vi "周围雷数.vi"(9 "列":dbl, 10 "行":dbl, 11 "雷区":dbl[][](array[numeric])) -> (3 "雷数":dbl)   [LabVIEW 2012]
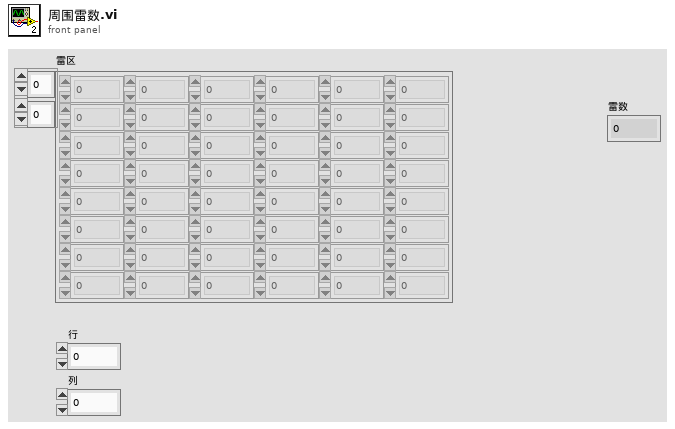
[diagram p1: front panel]
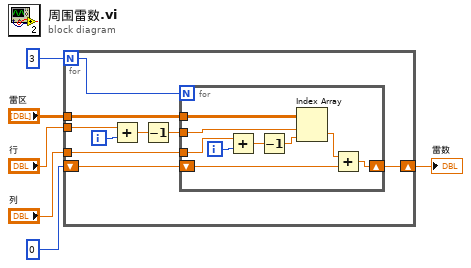
[diagram p0: block diagram]
diagram:
  n1 = for {
    N: 3 -> [w15]
    tunnel: "雷区" -> [w14]
    shift-right: [w7] -> w3
    shift-left: 0 -> [w13]
    tunnel: "行" -> [w10]
    tunnel: "列" -> [w12]
    i -> [w11]
    n2 = Add(x=w10, y=w11) -> (x+y=w9:dbl)
    n3 = Decrement(x=w9) -> (x-1=w8:dbl)
    n4 = for {
      N: w15 -> [_]
      tunnel: w14 -> [w21]
      shift-right: [w16] -> w7
      shift-left: w13 -> [w17]
      tunnel: w12 -> [w24]
      tunnel: w8 -> [w20]
      i -> [w23]
      n5 = Add(x=w24, y=w23) -> (x+y=w22:dbl)
      n6 = Decrement(x=w22) -> (x-1=w19:dbl)
      n7 = Index Array(array=w21, index (row)=w20, index (col)=w19) -> (element=w18:dbl)
      n8 = Add(x=w18, y=w17) -> (x+y=w16:dbl)
    }
  }
  "雷数" <- w3
